vi "labview code.vi"() -> ()   [LabVIEW 2019]
panel:
  out "set out one per time":string[](array[string])
  out "string array":string[](array[string])
  out "return value":string
  out "indata":string
  out "same qrcode?":bool
  out "Array":string[](array[string])
  in  "qrcode name":string
  out "DATA OUT = 1?":bool
  out "String s4":string
  out "String s3":string
  out "String s2":string
  out "state 3":string
  out "state 2":string
  out "state 1":string
  out "String s1":string
  out "state 4":string
  out "接收機械手臂工作狀態":string
  out "String":string
  in  "清除動作等待暫存器":bool
  out "result string":string
  out "DONE?":bool
  out "Numeric":i32
  in  "執行目標訂單\n的對應的動作":bool
  in  "清除訂單數據":bool
  out "對應訂單內容":string[](array[string])
  out "第幾項工作":string
  in  "要執行動作的訂單":string
  in  "nama Info":string[](array[string])
  in  "開始訂單系統":bool
  out "set out":set{string[]}(c389)
  out "訂單列表":string[][](array[string])
  out "element":string
  out "x = y?":bool
  in  "輸入區":T1
  in  "ZPZ":string="300"
  in  "ZPY":string="200"
  in  "ZPX":string="100"
  out "輸出資料查看列表":string[](array[string])
  out "DO number":u32
  in  "DO":bool[](array[boolean])
  in  "輸出資料初始值":string="{0,368,293.5,180,0,90}"
  in  "TO P0 2":bool
  out "輸出資料字串":string
  in  "stop":bool
  in  "Port":u16=5000
  in  "Service name":string="192.168.43.45"
  # "訂單系統"
  # "TCP連接"
  # "機械手臂數據"
types:
  T1 = cluster{"類別":string, "No.":string, "動作項目":string[], "輸入訂單":bool}
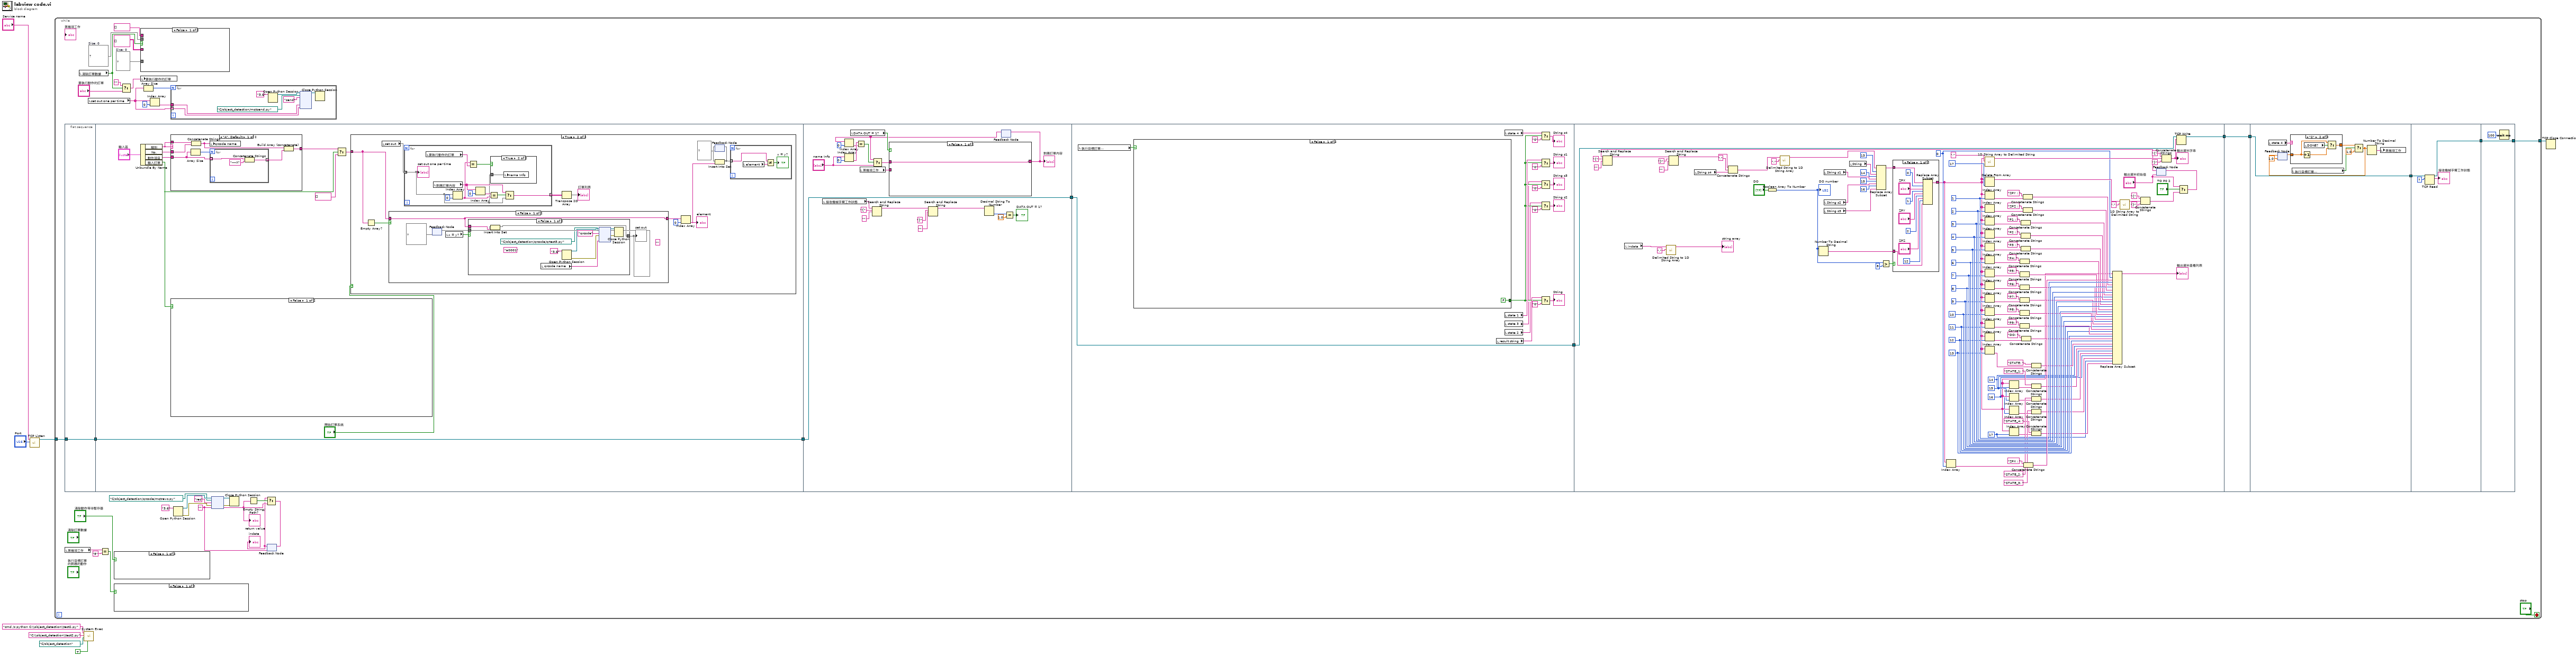
[diagram p0: block diagram]
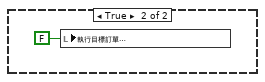
[diagram p2: hidden frame]
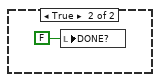
[diagram p3: hidden frame]
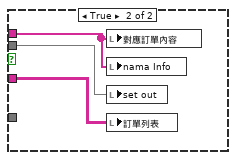
[diagram p4: hidden frame]
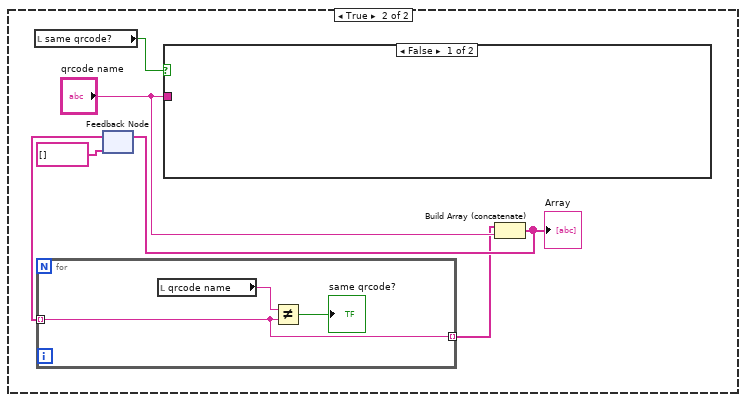
[diagram p5: hidden frame]
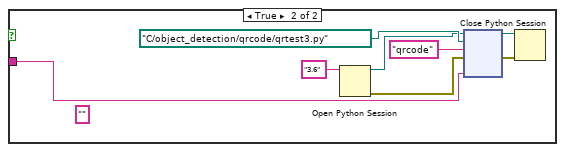
[diagram p6: hidden frame]
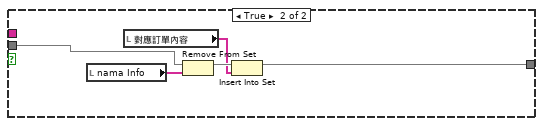
[diagram p9: hidden frame]
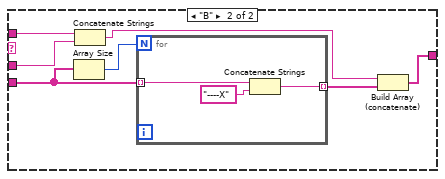
[diagram p11: hidden frame]
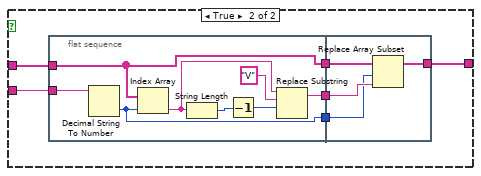
[diagram p12: hidden frame]
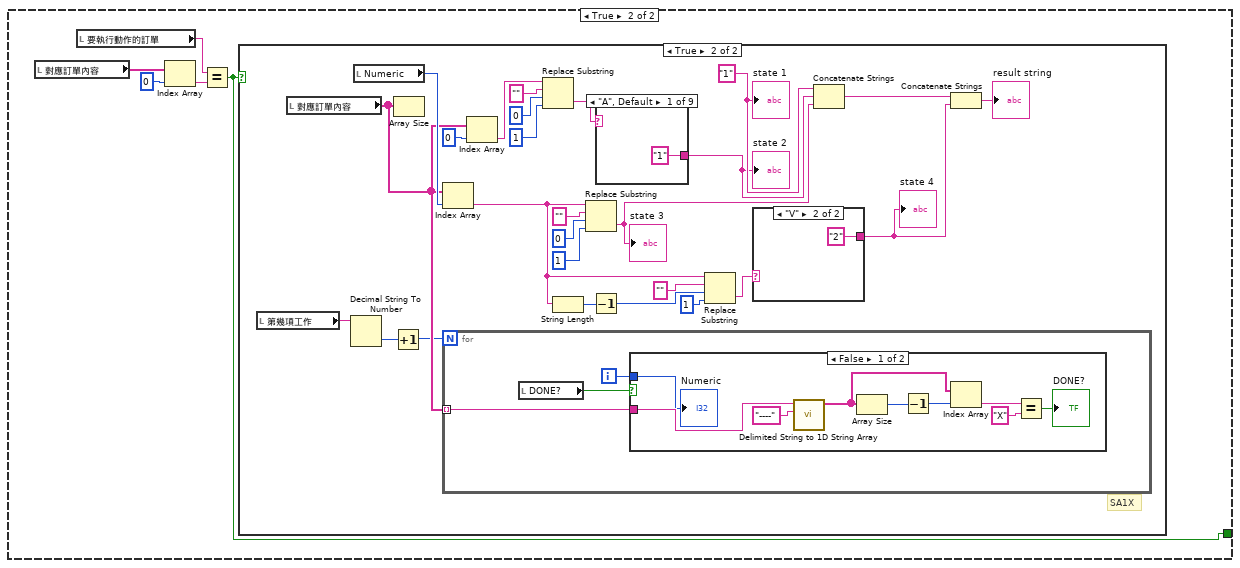
[diagram p13: hidden frame]
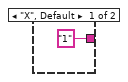
[diagram p15: hidden frame]
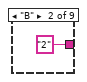
[diagram p16: hidden frame]
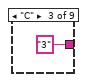
[diagram p17: hidden frame]
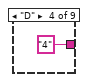
[diagram p18: hidden frame]
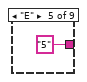
[diagram p19: hidden frame]
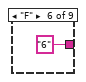
[diagram p20: hidden frame]
diagram:
  n1 = call <vilib>:"TCP Listen.vi"("port"="Port", "service name"="Service name") -> ("connection ID"=w8:refnum<k5>)  [unwired: 5 in, 4 out]
  n2 = while {
    tunnel: w8 -> [w46]
    tunnel: [w45] -> w7
    stop <- "stop" stop-if-true
    w17 = ""
    w37 = set{string} {}  # Size: 0
    w38 = set{string[]} {}  # Size: 0
    n3 = flat-sequence {
      tunnel: w46 -> [w60]
      tunnel: [w60] -> w25
      tunnel: [w70] -> w44
      tunnel: w25 -> [w70]
      tunnel: [w176] -> w35
      tunnel: w44 -> [w176]
      tunnel: w35 -> [w213]
      tunnel: [w213] -> w34
      tunnel: [w332] -> w27
      tunnel: w34 -> [w333]
      tunnel: w27 -> [w400]
      tunnel: [w400] -> w26
      tunnel: w26 -> [w409]
      tunnel: [w409] -> w33
      tunnel: w33 -> [w416]
      tunnel: [w415] -> w31
      tunnel: [w420] -> w45
      tunnel: w31 -> [w420]
      frame #0 {
      }
      frame #1 {
        n4 = Unbundle By Name("輸入區") -> ("類別"=w65:string, "No."=w64:string, "動作項目"=w66:string[], "輸入訂單"=w61:bool)
        n5 = case shown="\"A\", Default" w65 {
          tunnel: w64 -> [w140 w149]
          tunnel: w65 -> [w141 w150]
          tunnel: w66 -> [w137 w145]
          tunnel: [w139 w148] -> w68
          frame "A", Default {
            n6 = Array Size(array=w137) -> (size(s)=w138:i32)
            n7 = Concatenate Strings(w141, w140) -> (w135:string)
            n8 = local write "qrcode name"(w135) -> ()
            n9 = for {
              N: w138 -> [_]
              tunnel: w137 -> [w144] mode=indexing
              tunnel: [w142] -> w136 mode=indexing
              n10 = Concatenate Strings(w144, "----X") -> (w142:string)
            }
            n11 = Build Array (concatenate)(w135, w136) -> (w139:string[])
          }
          frame "B" {
            n12 = Array Size(array=w145) -> (size(s)=w147:i32)
            n13 = Concatenate Strings(w150, w149) -> (w151:string)
            n14 = for {
              N: w147 -> [_]
              tunnel: w145 -> [w154] mode=indexing
              tunnel: [w152] -> w146 mode=indexing
              n15 = Concatenate Strings(w154, "----X") -> (w152:string)
            }
            n16 = Build Array (concatenate)(w151, w146) -> (w148:string[])
          }
        }
        n17 = case shown="False" w61 {
          frame False {
          }
          frame True {
            n18 = local read "same qrcode?"() -> (w71:bool)
            n19 = feedback #1(string[] []) -> (w73:string[])
            n20 = for {
              tunnel: w73 -> [w78] mode=indexing
              tunnel: [w78] -> w72 mode=indexing
              n21 = local read "qrcode name"() -> (w79:string)
              n22 = Not Equal?(x=w79, y=w78) -> (x != y?=→"same qrcode?":bool)
            }
            n23 = case shown="False" w71 {
              tunnel: "qrcode name" -> [_ w80]
              frame False {
              }
              frame True {
                (unwired) ""
                n24 = Open Python Session(python version="3.6" ("Python version")) -> (session out=w82:refnum<k35>, error out=w84:errorcluster)  [unwired: 2 in]
                n25 = node(w82, path "C:/object_detection/qrcode/qrtest3.py" ("module path"), "qrcode" ("function name"), w84, w80) -> (w85:refnum<k35>, w86:errorcluster)  [unwired: 3 in, 2 out]
                n26 = Close Python Session(session in=w85, error in=w86) -> ()  [unwired: 1 out]
              }
            }
            n27 = Build Array (concatenate)(w72, "qrcode name") -> (w74:string[])
            "Array" <- w74
            n28 = feedback-in #1(w74) -> ()
          }
        }
        n29 = Select(t=w68, s=w61, f=string[] []) -> (s? t:f=w69:string[])
        n30 = case shown="True" "開始訂單系統" {
          tunnel: w69 -> [_ w98]
          frame False {
          }
          frame True {
            n31 = Empty Array?(array=w98) -> (empty?=w97:bool)
            n32 = local read "set out"() -> (w88:set{string[]})
            n33 = case shown="False" w97 {
              tunnel: w98 -> [w113 w134]
              tunnel: [w113 w134] -> w89
              frame False {
                (unwired) ""
                n34 = feedback #2(set{string[]} {} ("set in")) -> (w115:set{string[]})
                n35 = local read "x = y?"() -> (w117:bool)
                n36 = case shown="False" w117 {
                  tunnel: w115 -> [w127 w133]
                  tunnel: [w126 w130] -> w114
                  tunnel: w113 -> [w128 _]
                  frame False {
                    (unwired) "a0001"
                    n37 = Insert Into Set(10:w128, 11:w127) -> (3:w126:set{string[]})  [unwired: 1 out]
                    n38 = local read "qrcode name"() -> (w118:string)
                    n39 = Open Python Session(python version="3.6" ("Python version")) -> (session out=w125:refnum<k35>, error out=w124:errorcluster)  [unwired: 2 in]
                    n40 = node(w125, path "C:/object_detection/qrcode/qrtest3.py" ("module path"), "qrcode" ("function name"), w124, w118) -> (w123:refnum<k35>, w122:errorcluster)  [unwired: 3 in, 2 out]
                    n41 = Close Python Session(session in=w123, error in=w122) -> ()  [unwired: 1 out]
                  }
                  frame True {
                    n42 = local read "nama Info"() -> (w132:string[])
                    n43 = local read "對應訂單內容"() -> (w129:string[])
                    n44 = Remove From Set(10:w132, 11:w133) -> (3:w131:set{string[]})  [unwired: 1 out]
                    n45 = Insert Into Set(10:w129, 11:w131) -> (3:w130:set{string[]})  [unwired: 1 out]
                  }
                }
                "set out" <- w114
                n46 = feedback-in #2(w114) -> ()
              }
              frame True {
              }
            }
            n47 = for {
              tunnel: [w103] -> w95 mode=indexing
              tunnel: w88 -> [w102] mode=indexing
              n48 = local read "要執行動作的訂單"() -> (w109:string)
              n49 = local read "對應訂單內容"() -> (w104:string[])
              n50 = Index Array(array=w102, index=0) -> (element=w106:string)
              n51 = Equal?(x=w106, y=w109) -> (x = y?=w110:bool)
              n52 = Index Array(array=w104, index=0) -> (element=w107:string)
              n53 = Equal?(x=w107, y=w106) -> (x = y?=w105:bool)
              n54 = case shown="True" w110 {
                tunnel: w102 -> [_ w112]
                frame False {
                }
                frame True {
                  n55 = local write "nama Info"(w112) -> ()
                }
              }
              n56 = Select(t=w104, s=w105, f=w102) -> (s? t:f=w103:string[])
              "set out one per time" <- w102
            }
            n57 = Transpose 2D Array(2D array=w95) -> (transposed array=→"訂單列表":string[][])
            n58 = Index Array(array=w89, index=0) -> (element=w92:string)
            "element" <- w92
            n59 = feedback #3(set{string} {} ("set in")) -> (w94:set{string})
            n60 = Insert Into Set(10:w92, 11:w94) -> (3:w93:set{string})  [unwired: 1 out]
            n61 = feedback-in #3(w93) -> ()
            n62 = for {
              tunnel: w93 -> [w101] mode=indexing
              n63 = local read "element"() -> (w100:string)
              n64 = Not Equal?(x=w101, y=w100) -> (x != y?=→"x = y?":bool)
            }
          }
        }
      }
      frame #2 {
        n65 = local read "接收機械手臂工作狀態"() -> (w175:string)
        n66 = Index Array(array="nama Info", index=0) -> (element=w169:string)
        n67 = local read "DATA OUT = 1?"() -> (w170:bool)
        n68 = local read "第幾項工作"() -> (w162:string)
        n69 = Search and Replace String(input string=w175, search string="{", replace string="" ("replace string (\"\")")) -> (result string=w174:string)  [unwired: 5 in, 3 out]
        n70 = Search and Replace String(input string=w174, search string="}", replace string="" ("replace string (\"\")")) -> (result string=w171:string)  [unwired: 5 in, 3 out]
        n71 = Decimal String To Number(string=w171) -> (number=w173:i32)  [unwired: 2 in, 1 out]
        n72 = feedback #4() -> (w164:string[])  [unwired: 1 in]
        n73 = Index Array(array=w164, index=0) -> (element=w168:string)
        n74 = Equal?(x=w169, y=w168) -> (x = y?=w167:bool)
        n75 = Select(t=w164, s=w167, f="nama Info") -> (s? t:f=w166:string[])
        n76 = case shown="False" w170 {
          tunnel: w162 -> [_ w183]
          tunnel: w166 -> [w177 w182]
          tunnel: [w177 w181] -> w163
          frame False {
          }
          frame True {
            n77 = flat-sequence {
              tunnel: w183 -> [w187]
              tunnel: w182 -> [w186]
              tunnel: [w186] -> w180
              tunnel: [w185] -> w179
              tunnel: [w184] -> w178
              tunnel: [w192] -> w181
              tunnel: w180 -> [w193]
              tunnel: w179 -> [w195]
              tunnel: w178 -> [w194]
              frame #0 {
                n78 = Decimal String To Number(string=w187) -> (number=w184:i32)  [unwired: 2 in, 1 out]
                n79 = Index Array(array=w186, index=w184) -> (element=w191:string)
                n80 = String Length(string=w191) -> (length=w189:i32)
                n81 = Decrement(x=w189) -> (x-1=w190:i32)
                n82 = Replace Substring(3:w190, 4:"V" ("substring (\"\")"), 5:w191) -> (1:w185:string)  [unwired: 1 in, 1 out]
              }
              frame #1 {
                n83 = Replace Array Subset(array=w193, new element=w195, index=w194) -> (w192:string[])
              }
            }
          }
        }
        "對應訂單內容" <- w163
        n84 = feedback-in #4(w163) -> ()
        n85 = Equal?(x=w173, y=1.0) -> (x = y?=→"DATA OUT = 1?":bool)
      }
      frame #3 {
        n86 = local read "執行目標訂單\n的對應的動作"() -> (w212:bool)
        n87 = case shown="False" w212 {
          tunnel: [FALSE w215] -> w201
          frame False {
          }
          frame True {
            n88 = local read "對應訂單內容"() -> (w219:string[])
            n89 = local read "要執行動作的訂單"() -> (w217:string)
            n90 = Index Array(array=w219, index=0) -> (element=w216:string)
            n91 = Equal?(x=w217, y=w216) -> (x = y?=w215:bool)
            n92 = case shown="True" w215 {
              frame False {
              }
              frame True {
                w225 = "1" ("string")
                # "SA1X"
                n93 = local read "第幾項工作"() -> (w222:string)
                n94 = local read "對應訂單內容"() -> (w236:string[])
                n95 = Decimal String To Number(string=w222) -> (number=w221:i32)  [unwired: 2 in, 1 out]
                n96 = local read "Numeric"() -> (w237:i32)
                n97 = Increment(x=w221) -> (x+1=w220:i32)
                n98 = Array Size(array=w236) -> ()  [unwired: 1 out]
                n99 = Index Array "Index Array"(array=w236, index=w237) -> (element=w244:string)
                n100 = for {
                  N: w220 -> [_]
                  tunnel: w236 -> [w259] mode=indexing
                  i -> [w258]
                  n101 = local read "DONE?"() -> (w257:bool)
                  n102 = case shown="False" w257 {
                    tunnel: w259 -> [w266 _]
                    tunnel: w258 -> [w263 _]
                    frame False {
                      n103 = call <vilib>:"Delimited String to 1D String Array.vi"("delimiter"="----", "delimited string"=w266) -> ("string array"=w268:string[])  [unwired: 9 in]
                      n104 = Array Size(array=w268) -> (size(s)=w265:i32)
                      n105 = Decrement(x=w265) -> (x-1=w264:i32)
                      n106 = Index Array(array=w268, index=w264) -> (element=w262:string)
                      n107 = Equal?(x=w262, y="X") -> (x = y?=→"DONE?":bool)
                      "Numeric" <- w263
                    }
                    frame True {
                    }
                  }
                }
                n108 = Index Array(array=w236, index=0) -> (element=w232:string)
                n109 = Replace Substring(2:1 ("length (len. of substring)"), 3:0 ("offset (0)"), 4:"" ("substring (\"\")"), 5:w232) -> (0:w230:string)  [unwired: 1 out]
                n110 = String Length(string=w244) -> (length=w240:i32)
                n111 = Replace Substring(2:1 ("length (len. of substring)"), 3:0 ("offset (0)"), 4:"" ("substring (\"\")"), 5:w244) -> (0:w223:string)  [unwired: 1 out]
                "state 3" <- w223
                n112 = Decrement(x=w240) -> (x-1=w241:i32)
                n113 = case shown="\"A\", Default" w230 {
                  tunnel: ["1" "2" "3" "4" "5" "6" "7" "8" "9"] -> w224
                  frame "A", Default {
                  }
                  frame "B" {
                  }
                  frame "C" {
                  }
                  frame "D" {
                  }
                  frame "E" {
                  }
                  frame "F" {
                  }
                  frame "G" {
                  }
                  frame "H" {
                  }
                  frame "I" {
                  }
                }
                "state 2" <- w224
                n114 = Replace Substring(2:1 ("length (len. of substring)"), 3:w241, 4:"" ("substring (\"\")"), 5:w244) -> (0:w229:string)  [unwired: 1 out]
                n115 = case shown="\"V\"" w229 {
                  tunnel: ["1" "2"] -> w227
                  frame "X", Default {
                  }
                  frame "V" {
                  }
                }
                "state 4" <- w227
                n116 = Concatenate Strings(w225, w224, w223) -> (w228:string)
                n117 = Concatenate Strings(w228, w227) -> (→"result string":string)
                "state 1" <- w225
              }
            }
          }
        }
        n118 = local read "result string"() -> (w211:string)
        n119 = local read "state 4"() -> (w198:string)
        n120 = local read "state 1"() -> (w206:string)
        n121 = local read "state 3"() -> (w199:string)
        n122 = local read "state 2"() -> (w200:string)
        n123 = Select(t=w198, s=w201, f="0") -> (s? t:f=→"String s4":string)
        n124 = Select(t=w206, s=w201, f="0") -> (s? t:f=→"String s1":string)
        n125 = Select(t=w199, s=w201, f="0") -> (s? t:f=→"String s3":string)
        n126 = Select(t=w200, s=w201, f="0") -> (s? t:f=→"String s2":string)
        n127 = Select(t=w211, s=w201, f="0") -> (s? t:f=→"String":string)
      }
      frame #4 {
        w272 = 17 ("index")
        w274 = 16 ("index")
        w276 = 15 ("index")
        w291 = 14 ("index")
        w301 = 13 ("index")
        w308 = 12 ("index")
        w310 = 11 ("index")
        w316 = 10 ("index")
        w320 = 9 ("index")
        w322 = 8 ("index")
        w324 = 7 ("index")
        w335 = 6 ("index")
        w339 = 5 ("index")
        w342 = 4 ("index")
        w347 = 3 ("index")
        w350 = 2 ("index")
        w355 = 1 ("index")
        w362 = 0 ("index")
        n128 = local read "indata"() -> (w271:string)
        n129 = call <vilib>:"Delimited String to 1D String Array.vi"("delimiter"=",", "delimited string"=w271) -> ("string array"=→"string array":string[])  [unwired: 9 in]
        n130 = local read "String s4"() -> (w300:string)
        n131 = Boolean Array To Number(Boolean array="DO") -> (number=w307:u32)
        "DO number" <- w307
        n132 = Number To Decimal String(number=w307) -> (decimal integer string=w299:string)  [unwired: 1 in]
        n133 = local read "String s1"() -> (w290:string)
        n134 = local read "String s2"() -> (w289:string)
        n135 = local read "String s3"() -> (w288:string)
        n136 = local read "String"() -> (w296:string)
        n137 = Greater?(x=w307, y=u32 8) -> (0:w306:bool)
        n138 = feedback #5("輸出資料初始值") -> (w374:string)
        n139 = Search and Replace String(input string=w374, search string="{", replace string="" ("replace string (\"\")")) -> (result string=w382:string)  [unwired: 5 in, 3 out]
        n140 = Search and Replace String(input string=w382, search string="}", replace string="" ("replace string (\"\")")) -> (result string=w375:string)  [unwired: 5 in, 3 out]
        n141 = Concatenate Strings "Concatenate Strings"(w375, "," ("string"), w300) -> (w380:string)
        n142 = call <vilib>:"Delimited String to 1D String Array.vi"("delimiter"=",", "delimited string"=w380) -> ("string array"=w298:string[])  [unwired: 9 in]
        n143 = Replace Array Subset(array=w298, new element #1=w296, index #1=13 ("index"), new element #2=w290, index #2=14 ("index"), new element #3=w289, index #3=15 ("index"), new element #4=w288, index #4=16 ("index")) -> (w297:string[])
        n144 = case shown="False" w306 {
          tunnel: w297 -> [w392 w399]
          tunnel: [w391 w399] -> w278
          tunnel: w299 -> [w390 _]
          frame False {
            n145 = Replace Array Subset(array=w392, new element #1="ZPX", index #1=0 ("index"), new element #2="ZPY", index #2=1 ("index"), new element #3="ZPZ", index #3=2 ("index"), new element #4=w390, index #4=12 ("index")) -> (w391:string[])
          }
          frame True {
          }
        }
        n146 = Index Array "Index Array"(array=w278, index=w362) -> (element=w360:string)
        n147 = call <vilib>:"1D String Array to Delimited String.vi"("delimiter"=",", "string array"=w278) -> ("delimited string"=w378:string)  [unwired: 9 in]
        n148 = Delete From Array "Delete From Array"(array=w278, index=17) -> (array with subset deleted=w368:string[])  [unwired: 1 in, 1 out]
        n149 = Index Array(array=w278, index=w355) -> (element=w356:string)
        n150 = Index Array(array=w278, index=w350) -> (element=w352:string)
        n151 = Index Array(array=w278, index=w347) -> (element=w348:string)
        n152 = Index Array(array=w278, index=w342) -> (element=w344:string)
        n153 = Index Array(array=w278, index=w339) -> (element=w340:string)
        n154 = Index Array(array=w278, index=w335) -> (element=w336:string)
        n155 = Index Array(array=w278, index=w324) -> (element=w331:string)
        n156 = Index Array(array=w278, index=w322) -> (element=w330:string)
        n157 = Index Array(array=w278, index=w320) -> (element=w329:string)
        n158 = Index Array(array=w278, index=w316) -> (element=w319:string)
        n159 = Index Array(array=w278, index=w310) -> (element=w315:string)
        n160 = Index Array(array=w278, index=w308) -> (element=w314:string)
        n161 = Index Array(array=w278, index=w301) -> (element=w304:string)
        n162 = Index Array(array=w278, index=w291) -> (element=w294:string)
        n163 = Index Array(array=w278, index=w276) -> (element=w284:string)
        n164 = Index Array(array=w278, index=w274) -> (element=w282:string)
        n165 = Index Array(array=w278, index=w272) -> (element=w280:string)
        n166 = Concatenate Strings("P4: " ("string"), w336) -> (w334:string)
        n167 = Concatenate Strings("P5: " ("string"), w331) -> (w325:string)
        n168 = Concatenate Strings("P6: " ("string"), w330) -> (w323:string)
        n169 = Concatenate Strings("P7: " ("string"), w329) -> (w321:string)
        n170 = Concatenate Strings("P8: " ("string"), w319) -> (w317:string)
        n171 = Concatenate Strings("P9: " ("string"), w315) -> (w311:string)
        n172 = Concatenate Strings("P1 : " ("string"), w348) -> (w346:string)
        n173 = Concatenate Strings("P2 : " ("string"), w344) -> (w343:string)
        n174 = Concatenate Strings("P3 : " ("string"), w340) -> (w338:string)
        n175 = Concatenate Strings("DO: " ("string"), w314) -> (w309:string)
        n176 = Concatenate Strings("ZPY : " ("string"), w356) -> (w354:string)
        n177 = Concatenate Strings("ZPZ : " ("string"), w352) -> (w351:string)
        n178 = Concatenate Strings("ZPX : " ("string"), w360) -> (w359:string)
        n179 = Concatenate Strings("STATE: " ("string"), w304) -> (w302:string)
        n180 = Concatenate Strings("STATE_1: " ("string"), w294) -> (w292:string)
        n181 = Concatenate Strings("STATE_2: " ("string"), w284) -> (w277:string)
        n182 = Concatenate Strings("STATE_3: " ("string"), w282) -> (w275:string)
        n183 = Concatenate Strings("STATE_4: " ("string"), w280) -> (w273:string)
        n184 = Replace Array Subset "Replace Array Subset"(array=w278, new element #1=w359, index #1=w362, new element #2=w354, index #2=w355, new element #3=w351, index #3=w350, new element #4=w346, index #4=w347, new element #5=w343, index #5=w342, new element #6=w338, index #6=w339, new element #7=w334, index #7=w335, new element #8=w325, index #8=w324, new element #9=w323, index #9=w322, new element #10=w321, index #10=w320, new element #11=w317, index #11=w316, new element #12=w311, index #12=w310, new element #13=w309, index #13=w308, new element #14=w302, index #14=w301, new element #15=w292, index #15=w291, new element #16=w277, index #16=w276, new element #17=w275, index #17=w274, new element #18=w273, index #18=w272) -> (→"輸出資料查看列表":string[])
        n185 = call <vilib>:"1D String Array to Delimited String.vi"("delimiter"=",", "string array"=w368) -> ("delimited string"=w371:string)  [unwired: 9 in]
        n186 = Concatenate Strings("{" ("string"), w371, "}" ("string")) -> (w365:string)
        n187 = Concatenate Strings("{" ("string"), w378, "}" ("string")) -> (w366:string)
        "輸出資料字串" <- w366
        n188 = TCP Write(connection ID=w333, data in=w366) -> (connection ID out=w332:refnum<k5>)  [unwired: 2 in, 2 out]
        n189 = Select(t="輸出資料初始值", s="TO P0 2", f=w365) -> (s? t:f=w364:string)
        n190 = feedback-in #5(w364) -> ()
      }
      frame #5 {
      }
      frame #6 {
        n191 = local read "state 4"() -> (w403:string)
        n192 = feedback #6(1.0 ("t")) -> (w404:dbl)
        n193 = case shown="\"2\"" w403 {
          tunnel: w404 -> [w410 w411]
          tunnel: [w410 w413] -> w407
          frame "1", Default {
          }
          frame "2" {
            n194 = Increment(x=w411) -> (x+1=w412:dbl)
            n195 = local read "DONE?"() -> (w414:bool)
            n196 = Select(t=w411, s=w414, f=w412) -> (s? t:f=w413:dbl)
          }
        }
        n197 = local read "執行目標訂單\n的對應的動作"() -> (w406:bool)
        n198 = Select(t=w407, s=w406, f=1.0) -> (s? t:f=w408:dbl)
        n199 = feedback-in #6(w408) -> ()
        n200 = Number To Decimal String(number=w408) -> (decimal integer string=w405:string)  [unwired: 1 in]
        n201 = local write "第幾項工作"(w405) -> ()
      }
      frame #7 {
        n202 = TCP Read(connection ID=w416, bytes to read=7) -> (connection ID out=w415:refnum<k5>, data out=→"接收機械手臂工作狀態":string)  [unwired: 3 in, 1 out]
      }
      frame #8 {
        n203 = Wait (ms)(milliseconds to wait=u32 100) -> ()  [unwired: 1 out]
      }
    }
    n204 = local read "第幾項工作"() -> (w30:string)
    n205 = local read "清除訂單數據"() -> (w41:bool)
    n206 = local read "set out one per time"() -> (w10:string[])
    n207 = Equal?(x=w30, y="5") -> (x = y?=w28:bool)
    n208 = case shown="False" "清除動作等待暫存器" {
      frame False {
      }
      frame True {
        n209 = local write "DONE?"(FALSE) -> ()
      }
    }
    n210 = case shown="False" w28 {
      frame False {
      }
      frame True {
        n211 = local write "執行目標訂單\n的對應的動作"(FALSE) -> ()
      }
    }
    n212 = Select(t="", s=w41, f="要執行動作的訂單") -> (s? t:f=w43:string)
    n213 = case shown="False" w41 {
      tunnel: string[] [] -> [_ w57]
      tunnel: w38 -> [_ w59]
      tunnel: w37 -> [_ _]
      tunnel: string[][] [] ("transposed array") -> [_ w58]
      frame False {
      }
      frame True {
        n214 = local write "對應訂單內容"(w57) -> ()
        n215 = local write "nama Info"(w57) -> ()
        n216 = local write "set out"(w59) -> ()
        n217 = local write "訂單列表"(w58) -> ()
      }
    }
    n218 = local write "要執行動作的訂單"(w43) -> ()
    n219 = Array Size(array=w10) -> (size(s)=w11:i32)
    n220 = Index Array(array=w10, index=0) -> (element=w9:string)
    n221 = for {
      N: w11 -> [_]
      tunnel: w10 -> [w48] mode=indexing
      tunnel: w9 -> [w49]
      n222 = Open Python Session(python version="3.6" ("Python version")) -> (session out=w54:refnum<k35>)  [unwired: 2 in, 1 out]
      n223 = node(w54, path "C:/object_detection/mqtsend.py" ("module path"), "send" ("function name"), w49, w48) -> (w53:refnum<k35>)  [unwired: 5 in, 3 out]
      n224 = Close Python Session(session in=w53) -> ()  [unwired: 1 in, 1 out]
    }
    n225 = Open Python Session(python version="3.6" ("Python version")) -> (session out=w24:refnum<k35>, error out=w23:errorcluster)  [unwired: 2 in]
    n226 = node(w24, path "C:/object_detection/qrcode/mqtrevc.py" ("module path"), "rec" ("function name"), w23, w17) -> (w22:refnum<k35>, w21:errorcluster, w19:string)  [unwired: 2 out]
    "return value" <- w19
    n227 = Close Python Session(session in=w22, error in=w21) -> ()  [unwired: 1 out]
    n228 = Empty String/Path?(string/path=w19) -> (empty?=w20:bool)
    n229 = feedback #7(w17) -> (w18:string)
    "indata" <- w18
    n230 = Select(t=w18, s=w20, f=w19) -> (s? t:f=w13:string)
    n231 = feedback-in #7(w13) -> ()
  }
  n232 = call <vilib>:"System Exec.vi"("run minimized? (F)"=TRUE, "working directory"=path "C:/object_detection", "standard input"="C:\\object_detection\\test2.py", "command line"="cmd /c python C:\\object_detection\\test2.py") -> ()  [unwired: 4 in, 4 out]
  n233 = TCP Close Connection(connection ID=w7) -> ()  [unwired: 2 in, 2 out]
